vi "Error Handler.vi"(8 "error in (no error)":errorcluster, 11 "Error_Control":T1) -> (0 "error out":errorcluster)   [LabVIEW 2013]
doc: "Error Handler. Interprets error conditions, logs errors, and sends commands back to the controller. The error type is set by the caller, the FGV responds depending on the error type."
uses:
  Error_Control.ctl
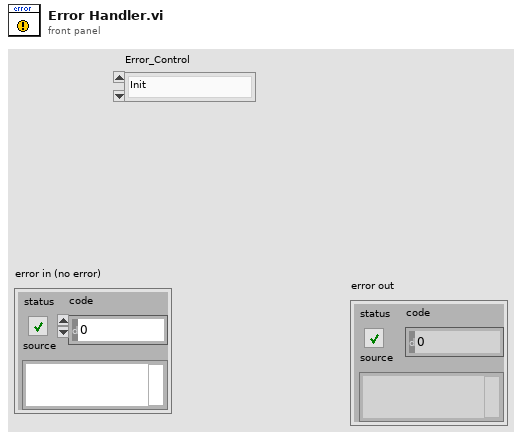
[diagram p1: front panel]
types:
  T1 = typedef "Error_Control.ctl" = enum16{"Init", "Console_err", "Process_err", "Sensor_err"}
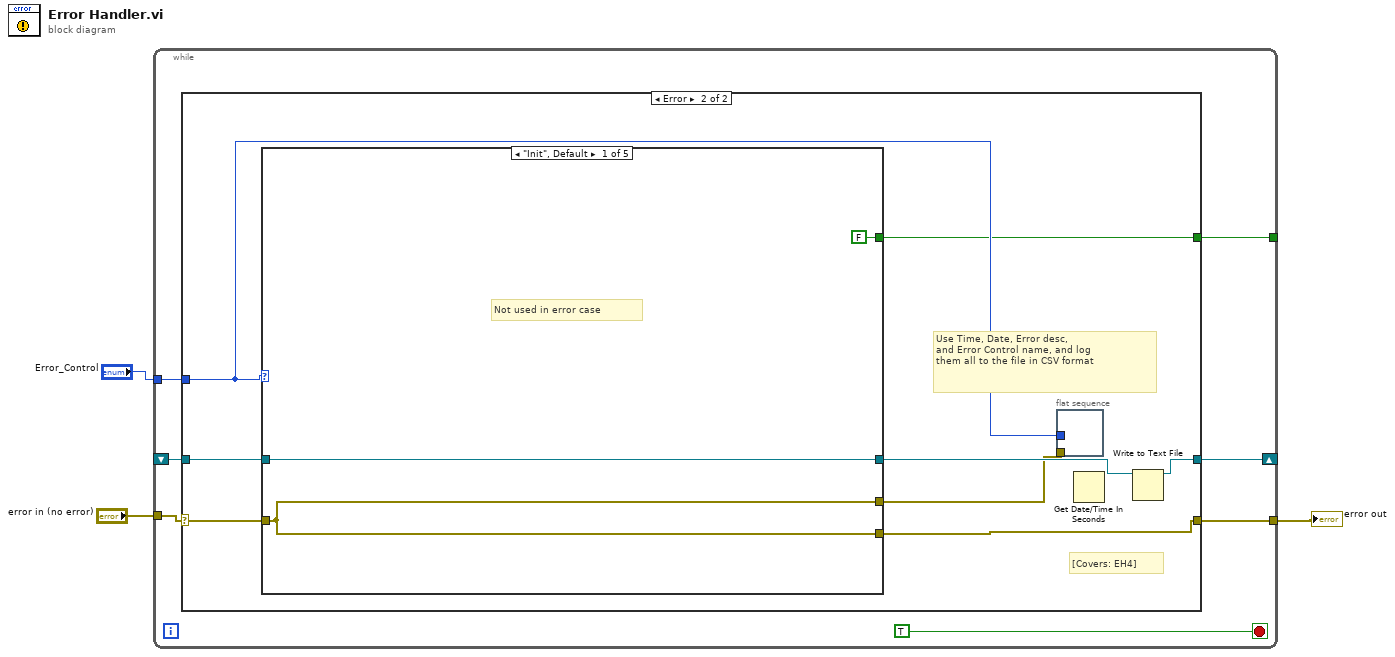
[diagram p0: block diagram]
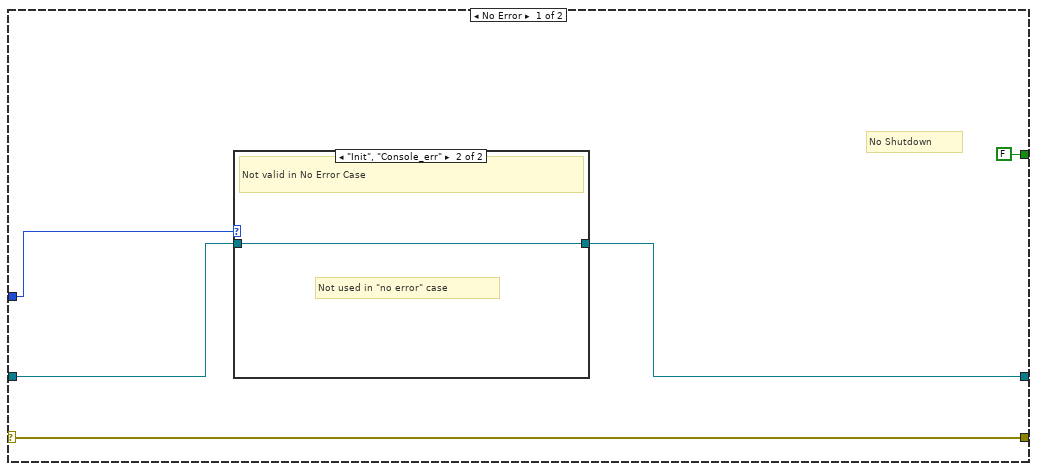
[diagram p2: hidden frame]
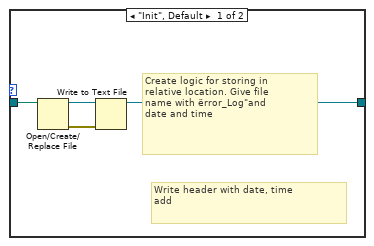
[diagram p3: hidden frame]
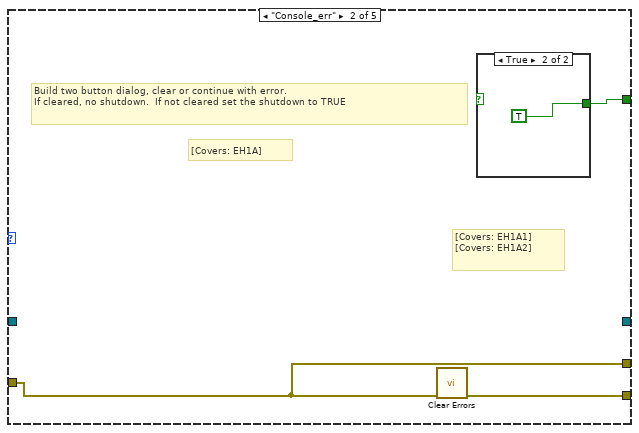
[diagram p4: hidden frame]
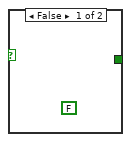
[diagram p5: hidden frame]
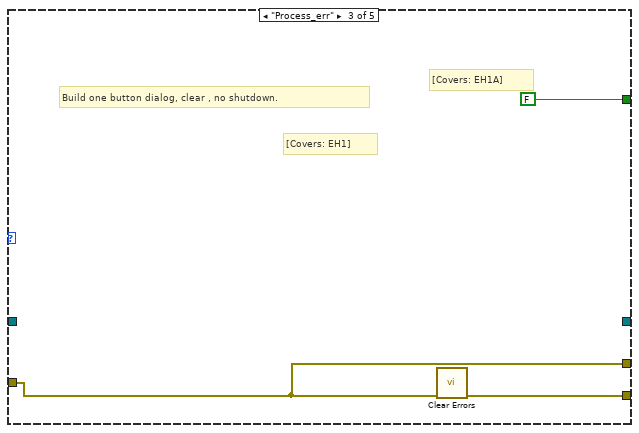
[diagram p6: hidden frame]
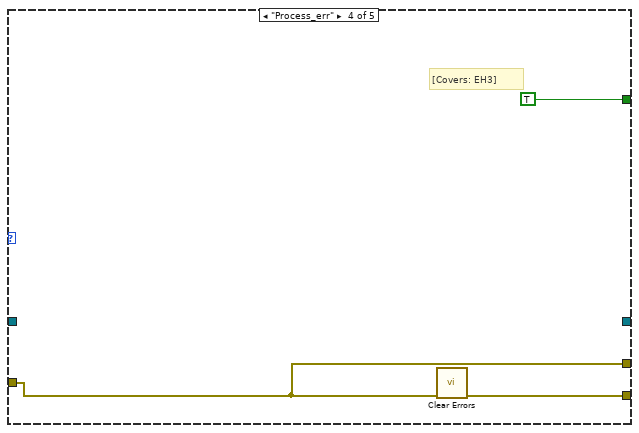
[diagram p7: hidden frame]
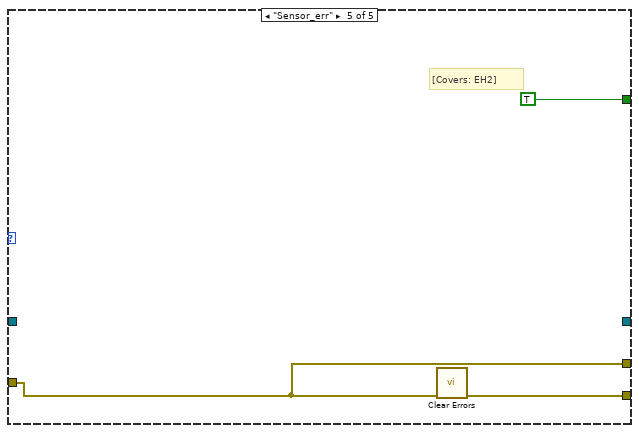
[diagram p8: hidden frame]
diagram:
  n1 = while {
    tunnel: "Error_Control" -> [w9]
    shift-right: [w8] -> _
    shift-left: _ -> [w6]
    tunnel: "error in (no error)" -> [w7]
    tunnel: [w5] -> w1
    tunnel: [w4] -> _
    stop <- TRUE stop-if-true
    n2 = case shown="Error" w7 {
      selector: w7 -> [w15 w25]
      tunnel: w9 -> [w14 w23]
      tunnel: [w12 w28] -> w8
      tunnel: w6 -> [w13 w26]
      tunnel: [w15 w24] -> w5
      tunnel: [FALSE w21] -> w4
      frame No Error {
        # "No Shutdown"
        n3 = case shown="\"Sensor_err\"..\"console_err\"" w14 {
          tunnel: [w17 w20] -> w12
          tunnel: w13 -> [_ w20]
          frame "Init", Default {
            # "Write header with date, time\nadd"
            # "Create logic for storing in\nrelative location. Give file\nname with ërror_Log\"and\ndate and time"
            n4 = Open/Create/Replace File(file path (use dialog)=path "") -> (refnum out=w18:refnum<file>, error out=w19:errorcluster)  [unwired: 5 in, 1 out]
            n5 = Write to Text File(file (use dialog)=w18, error in=w19) -> (refnum out=w17:refnum<file>)  [unwired: 2 in, 2 out]
          }
          frame "Init", "Console_err" {
            # "Not used in \"no error\" case"
            # "Not valid in No Error Case"
          }
        }
      }
      frame Error {
        # "[Covers: EH4]"
        # "Use Time, Date, Error desc, \nand Error Control name, and log \nthem all to the file in CSV format"
        n6 = case shown="\"Init\", Default" w23 {
          tunnel: [w30 _ _ _ _] -> w27
          tunnel: w26 -> [w30 _ _ _ _]
          tunnel: w25 -> [w31 w34 w38 w41 w44]
          tunnel: [w31 w33 w37 w40 w43] -> w24
          tunnel: [w31 w34 w38 w41 w44] -> w22
          tunnel: [FALSE w32 FALSE TRUE TRUE] -> w21
          frame "Init", Default {
            # "Not used in error case"
          }
          frame "Console_err" {
            # "[Covers: EH1A1]\n[Covers: EH1A2]"
            # "[Covers: EH1A]"
            # "Build two button dialog, clear or continue with error.\nIf cleared, no shutdown.  If not cleared set the shutdown to TRUE"
            n7 = call <vilib>:"Clear Errors.vi"("error in (no error)"=w34) -> ("error out"=w33:errorcluster)  [unwired: 6 in]
            n8 = case shown="True" {
              selector: _ -> [_ _]
              tunnel: [_ TRUE] -> w32
              frame False {
                (unwired) FALSE
              }
              frame True {
              }
            }
          }
          frame "Process_err" {
            # "[Covers: EH1]"
            # "[Covers: EH1A]"
            # "Build one button dialog, clear , no shutdown."
            n9 = call <vilib>:"Clear Errors.vi"("error in (no error)"=w38) -> ("error out"=w37:errorcluster)  [unwired: 6 in]
          }
          frame "Process_err" {
            # "[Covers: EH3]"
            n10 = call <vilib>:"Clear Errors.vi"("error in (no error)"=w41) -> ("error out"=w40:errorcluster)  [unwired: 6 in]
          }
          frame "Sensor_err" {
            # "[Covers: EH2]"
            n11 = call <vilib>:"Clear Errors.vi"("error in (no error)"=w44) -> ("error out"=w43:errorcluster)  [unwired: 6 in]
          }
        }
        n12 = flat-sequence {
          tunnel: w23 -> [_]
          tunnel: w22 -> [_]
          frame #0 {
          }
        }
        n13 = Get Date/Time In Seconds() -> ()  [unwired: 1 out]
        n14 = Write to Text File(file (use dialog)=w27) -> (refnum out=w28:refnum<file>)  [unwired: 3 in, 2 out]
      }
    }
  }
  "error out" <- w1
